vi "IRC5ControlViaOPC.vi"() -> ()   [LabVIEW 2019]
uses:
  <vilib>/OPCUA/controls/NodeId.ctl
  <vilib>/OPCUA/controls/Write Status.ctl
  <vilib>/OPCUA/controls/NodeIds.ctl
  <vilib>/OPCUA/controls/OPC UA StatusCode.ctl
  <vilib>/numeric/Random Number (Range) U64.vi
  <vilib>/numeric/sub_Random U32.vi
  <vilib>/OPCUA/client/Multiple Read Bool.vi
  <vilib>/OPCUA/client/Multiple Write Bool.vi
  <vilib>/OPCUA/NI OPC UA Client.lvlib
panel:
  in  "username/password":cluster{"username":string, "password":string}
  in  "Start":bool
  out "Color Box 45":u32(colorbox)
  out "Color Box 44":u32(colorbox)
  out "Color Box 43":u32(colorbox)
  out "Color Box 42":u32(colorbox)
  out "Color Box 41":u32(colorbox)
  out "Color Box 40":u32(colorbox)
  out "Color Box 39":u32(colorbox)
  out "Color Box 38":u32(colorbox)
  out "Color Box 37":u32(colorbox)
  out "Color Box 36":u32(colorbox)
  out "Color Box 35":u32(colorbox)
  out "Color Box 34":u32(colorbox)
  out "Color Box 33":u32(colorbox)
  out "Color Box 32":u32(colorbox)
  out "Color Box 31":u32(colorbox)
  out "Color Box 30":u32(colorbox)
  out "Color Box 29":u32(colorbox)
  out "Color Box 28":u32(colorbox)
  out "Color Box 27":u32(colorbox)
  out "Color Box 26":u32(colorbox)
  out "Color Box 25":u32(colorbox)
  out "Color Box 24":u32(colorbox)
  out "Color Box 23":u32(colorbox)
  out "Color Box 22":u32(colorbox)
  out "Color Box 21":u32(colorbox)
  out "Color Box 20":u32(colorbox)
  out "Color Box 19":u32(colorbox)
  out "Color Box 18":u32(colorbox)
  out "Color Box 12":u32(colorbox)
  out "Color Box 6":u32(colorbox)
  out "Color Box 17":u32(colorbox)
  out "Color Box 16":u32(colorbox)
  out "Color Box 15":u32(colorbox)
  out "Color Box 14":u32(colorbox)
  out "Color Box 13":u32(colorbox)
  out "Color Box 11":u32(colorbox)
  out "Color Box 10":u32(colorbox)
  out "Color Box 9":u32(colorbox)
  out "Color Box 8":u32(colorbox)
  out "Color Box 7":u32(colorbox)
  out "Color Box 5":u32(colorbox)
  out "Color Box 4":u32(colorbox)
  out "Color Box 3":u32(colorbox)
  out "Color Box 2":u32(colorbox)
  out "Color Box":u32(colorbox)
  out "Praca robota":bool
  out "element2":u32(colorbox)
  out "Układanie na palecie 3":bool
  out "Układanie na palecie 2":bool
  out "Układanie na palecie 1":bool
  out "Wrzucanie do kosza":bool
  out "Ilość elementów na palecie 1":dbl
  in  "Kolor na palecie 3":u16(ring) items=["czerwony", "zielony", "niebieski", "zółty", ""]
  in  "Kolor na palecie 2":u16(ring) items=["czerwony", "zielony", "niebieski", "zółty", ""]
  in  "Kolor na palecie 1":u16(ring) items=["czerwony", "zielony", "niebieski", "zółty", ""]
  in  "Kolor w koszu":u16(ring) items=["czerwony", "zielony", "niebieski", "zółty", ""]
  in  "milliseconds to wait 2":u32
  in  "milliseconds to wait":u32
  out "element":u32(colorbox)
  out "Ilość elementów na palecie 3":dbl
  out "Ilość elementów na palecie 2":dbl
  out "Ilość elementów w koszu":dbl
  out "Koniec przejazdu":bool
  out "Przejazd na przenośniku":bool
  out "Aktualny kolor":string
  in  "Sposób wyboru kolorów":enum32{"Losowanie", "Manualny Wybór"}(tab)
  out "Losowany kolor":string
  in  "Częstotliwość":dbl
  in  "Radio Buttons":enum32{"1", "2", "3", "4"}(radio)
  out "results":T3(array[cluster]) {"status" items=["Good"=0, "Good_SubscriptionTransferred"=2949120, "Good_CompletesAsynchronously"=3014656, "Good_Overload"=3080192, "Good_Clamped"=3145728, "Good_LocalOverride"=9830400, "Good_EntryInserted"=10616832, "Good_EntryReplaced"=10682368, "Good_NoData"=10813440, "Good_MoreData"=10878976, "Good_CommunicationEvent"=10944512, "Good_ShutdownEvent"=11010048, "Good_CallAgain"=11075584, "Good_NonCriticalTimeout"=11141120, "Good_ResultsMayBeIncomplete"=12189696, "Good_DataIgnored"=14221312, "Uncertain"=1073741824, "Uncertain_ReferenceOutOfServer"=1080819712, "Uncertain_NoCommunicationLastUsableValue"=1083113472, "Uncertain_LastUsableValue"=1083179008, "Uncertain_SubstituteValue"=1083244544, "Uncertain_InitialValue"=1083310080, "Uncertain_SensorNotAccurate"=1083375616, "Uncertain_EngineeringUnitsExceeded"=1083441152, "Uncertain_SubNormal"=1083506688, "Uncertain_DataSubNormal"=1084489728, "Uncertain_ReferenceNotDeleted"=1086062592, "Uncertain_NotAllNodesAvailable"=1086324736, "Bad"=2147483648, "Bad_UnexpectedError"=2147549184, "Bad_InternalError"=2147614720, "Bad_OutOfMemory"=2147680256, "Bad_ResourceUnavailable"=2147745792, "Bad_CommunicationError"=2147811328, "Bad_EncodingError"=2147876864, "Bad_DecodingError"=2147942400, "Bad_EncodingLimitsExceeded"=2148007936, "Bad_UnknownResponse"=2148073472, "Bad_Timeout"=2148139008, "Bad_ServiceUnsupported"=2148204544, "Bad_Shutdown"=2148270080, "Bad_ServerNotConnected"=2148335616, "Bad_ServerHalted"=2148401152, "Bad_NothingToDo"=2148466688, "Bad_TooManyOperations"=2148532224, "Bad_DataTypeIdUnknown"=2148597760, "Bad_CertificateInvalid"=2148663296, "Bad_SecurityChecksFailed"=2148728832, "Bad_CertificateTimeInvalid"=2148794368, "Bad_CertificateIssuerTimeInvalid"=2148859904, "Bad_CertificateHostNameInvalid"=2148925440, "Bad_CertificateUriInvalid"=2148990976, "Bad_CertificateUseNotAllowed"=2149056512, "Bad_CertificateIssuerUseNotAllowed"=2149122048, "Bad_CertificateUntrusted"=2149187584, "Bad_CertificateRevocationUnknown"=2149253120, "Bad_CertificateIssuerRevocationUnknown"=2149318656, "Bad_CertificateRevoked"=2149384192, "Bad_CertificateIssuerRevoked"=2149449728, "Bad_UserAccessDenied"=2149515264, "Bad_IdentityTokenInvalid"=2149580800, "Bad_IdentityTokenRejected"=2149646336, "Bad_SecureChannelIdInvalid"=2149711872, "Bad_InvalidTimestamp"=2149777408, "Bad_NonceInvalid"=2149842944, "Bad_SessionIdInvalid"=2149908480, "Bad_SessionClosed"=2149974016, "Bad_SessionNotActivated"=2150039552, "Bad_SubscriptionIdInvalid"=2150105088, "Bad_RequestHeaderInvalid"=2150236160, "Bad_TimestampsToReturnInvalid"=2150301696, "Bad_RequestCancelledByClient"=2150367232, "Bad_NoCommunication"=2150694912, "Bad_WaitingForInitialData"=2150760448, "Bad_NodeIdInvalid"=2150825984, "Bad_NodeIdUnknown"=2150891520, "Bad_AttributeIdInvalid"=2150957056, "Bad_IndexRangeInvalid"=2151022592, "Bad_IndexRangeNoData"=2151088128, "Bad_DataEncodingInvalid"=2151153664, "Bad_DataEncodingUnsupported"=2151219200, "Bad_NotReadable"=2151284736, "Bad_NotWritable"=2151350272, "Bad_OutOfRange"=2151415808, "Bad_NotSupported"=2151481344, "Bad_NotFound"=2151546880, "Bad_ObjectDeleted"=2151612416, "Bad_NotImplemented"=2151677952, "Bad_MonitoringModeInvalid"=2151743488, "Bad_MonitoredItemIdInvalid"=2151809024, "Bad_MonitoredItemFilterInvalid"=2151874560, "Bad_MonitoredItemFilterUnsupported"=2151940096, "Bad_FilterNotAllowed"=2152005632, "Bad_StructureMissing"=2152071168, "Bad_EventFilterInvalid"=2152136704, "Bad_ContentFilterInvalid"=2152202240, "Bad_FilterOperandInvalid"=2152267776, "Bad_ContinuationPointInvalid"=2152333312, "Bad_NoContinuationPoints"=2152398848, "Bad_ReferenceTypeIdInvalid"=2152464384, "Bad_BrowseDirectionInvalid"=2152529920, "Bad_NodeNotInView"=2152595456, "Bad_ServerUriInvalid"=2152660992, "Bad_ServerNameMissing"=2152726528, "Bad_DiscoveryUrlMissing"=2152792064, "Bad_SempahoreFileMissing"=2152857600, "Bad_RequestTypeInvalid"=2152923136, "Bad_SecurityModeRejected"=2152988672, "Bad_SecurityPolicyRejected"=2153054208, "Bad_TooManySessions"=2153119744, "Bad_UserSignatureInvalid"=2153185280, "Bad_ApplicationSignatureInvalid"=2153250816, "Bad_NoValidCertificates"=2153316352, "Bad_RequestCancelledByRequest"=2153381888, "Bad_ParentNodeIdInvalid"=2153447424, "Bad_ReferenceNotAllowed"=2153512960, "Bad_NodeIdRejected"=2153578496, "Bad_NodeIdExists"=2153644032, "Bad_NodeClassInvalid"=2153709568, "Bad_BrowseNameInvalid"=2153775104, "Bad_BrowseNameDuplicated"=2153840640, "Bad_NodeAttributesInvalid"=2153906176, "Bad_TypeDefinitionInvalid"=2153971712, "Bad_SourceNodeIdInvalid"=2154037248, "Bad_TargetNodeIdInvalid"=2154102784, "Bad_DuplicateReferenceNotAllowed"=2154168320, "Bad_InvalidSelfReference"=2154233856, "Bad_ReferenceLocalOnly"=2154299392, "Bad_NoDeleteRights"=2154364928, "Bad_ServerIndexInvalid"=2154430464, "Bad_ViewIdUnknown"=2154496000, "Bad_TooManyMatches"=2154627072, "Bad_QueryTooComplex"=2154692608, "Bad_NoMatch"=2154758144, "Bad_MaxAgeInvalid"=2154823680, "Bad_HistoryOperationInvalid"=2154889216, "Bad_HistoryOperationUnsupported"=2154954752, "Bad_WriteNotSupported"=2155020288, "Bad_TypeMismatch"=2155085824, "Bad_MethodInvalid"=2155151360, "Bad_ArgumentsMissing"=2155216896, "Bad_TooManySubscriptions"=2155282432, "Bad_TooManyPublishRequests"=2155347968, "Bad_NoSubscription"=2155413504, "Bad_SequenceNumberUnknown"=2155479040, "Bad_MessageNotAvailable"=2155544576, "Bad_InsufficientClientProfile"=2155610112, "Bad_TcpServerTooBusy"=2155675648, "Bad_TcpMessageTypeInvalid"=2155741184, "Bad_TcpSecureChannelUnknown"=2155806720, "Bad_TcpMessageTooLarge"=2155872256, "Bad_TcpNotEnoughResources"=2155937792, "Bad_TcpInternalError"=2156003328, "Bad_TcpEndpointUrlInvalid"=2156068864, "Bad_RequestInterrupted"=2156134400, "Bad_RequestTimeout"=2156199936, "Bad_SecureChannelClosed"=2156265472, "Bad_SecureChannelTokenUnknown"=2156331008, "Bad_SequenceNumberInvalid"=2156396544, "Bad_ConfigurationError"=2156462080, "Bad_NotConnected"=2156527616, "Bad_DeviceFailure"=2156593152, "Bad_SensorFailure"=2156658688, "Bad_OutOfService"=2156724224, "Bad_DeadbandFilterInvalid"=2156789760, "Bad_RefreshInProgress"=2157379584, "Bad_ConditionAlreadyDisabled"=2157445120, "Bad_ConditionDisabled"=2157510656, "Bad_EventIdUnknown"=2157576192, "Bad_NoData"=2157641728, "Bad_DataLost"=2157772800, "Bad_DataUnavailable"=2157838336, "Bad_EntryExists"=2157903872, "Bad_NoEntryExists"=2157969408, "Bad_TimestampNotSupported"=2158034944, "Bad_InvalidArgument"=2158690304, "Bad_ConnectionRejected"=2158755840, "Bad_Disconnect"=2158821376, "Bad_ConnectionClosed"=2158886912, "Bad_InvalidState"=2158952448, "Bad_EndOfStream"=2159017984, "Bad_NoDataAvailable"=2159083520, "Bad_WaitingForResponse"=2159149056, "Bad_OperationAbandoned"=2159214592, "Bad_ExpectedStreamToBlock"=2159280128, "Bad_WouldBlock"=2159345664, "Bad_SyntaxError"=2159411200, "Bad_MaxConnectionsReached"=2159476736, "Bad_RequestTooLarge"=2159542272, "Bad_ResponseTooLarge"=2159607808, "Bad_EventNotAcknowledgeable"=2159738880, "Bad_InvalidTimestampArgument"=2159869952, "Bad_ProtocolVersionUnsupported"=2159935488, "Bad_StateNotActive"=2160001024, "Bad_FilterOperatorInvalid"=2160132096, "Bad_FilterOperatorUnsupported"=2160197632, "Bad_FilterOperandCountMismatch"=2160263168, "Bad_FilterElementInvalid"=2160328704, "Bad_FilterLiteralInvalid"=2160394240, "Bad_IdentityChangeNotSupported"=2160459776, "Bad_NotTypeDefinition"=2160590848, "Bad_ViewTimestampInvalid"=2160656384, "Bad_ViewParameterMismatch"=2160721920, "Bad_ViewVersionInvalid"=2160787456, "Bad_ConditionAlreadyEnabled"=2160852992, "Bad_DialogNotActive"=2160918528, "Bad_DialogResponseInvalid"=2160984064, "Bad_ConditionBranchAlreadyAcked"=2161049600, "Bad_ConditionBranchAlreadyConfirmed"=2161115136, "Bad_ConditionAlreadyShelved"=2161180672, "Bad_ConditionNotShelved"=2161246208, "Bad_ShelvingTimeOutOfRange"=2161311744, "Bad_AggregateListMismatch"=2161377280, "Bad_AggregateNotSupported"=2161442816, "Bad_AggregateInvalidInputs"=2161508352, "Bad_BoundNotFound"=2161573888, "Bad_BoundNotSupported"=2161639424, "Bad_AggregateConfigurationRejected"=2161770496, "Bad_TooManyMonitoredItems"=2161836032]}
  in  "node IDs":T4
  in  "requests":T6(array[cluster]) {"node status" items=["Good"=0, "Uncertain"=1073741824, "Uncertain_InitialValue"=1083310080, "Uncertain_LastUsableValue"=1083179008, "Uncertain_SensorNotAccurate"=1083375616, "Uncertain_EngineeringUnitsExceeded"=1083441152, "Bad"=2147483648, "Bad_NoCommunication"=2150694912, "Bad_NotReadable"=2151284736, "Bad_NotWritable"=2151350272, "Bad_OutOfRange"=2151415808, "Bad_WaitingForInitialData"=2150760448]}
  in  "client certificate file":path
  in  "security policy":T7
  in  "stop":bool
  in  "trust any server (F)":bool
  in  "server endpoint URL":string
  # "Konfigutracja OPC CLIENT"
  # "Sterowanie procesem"
  # "Wizualizacja procesu"
  # "Paleta nr3"
  # "Sterowanie programem"
  # "Paleta nr1"
  # "Paleta nr2"
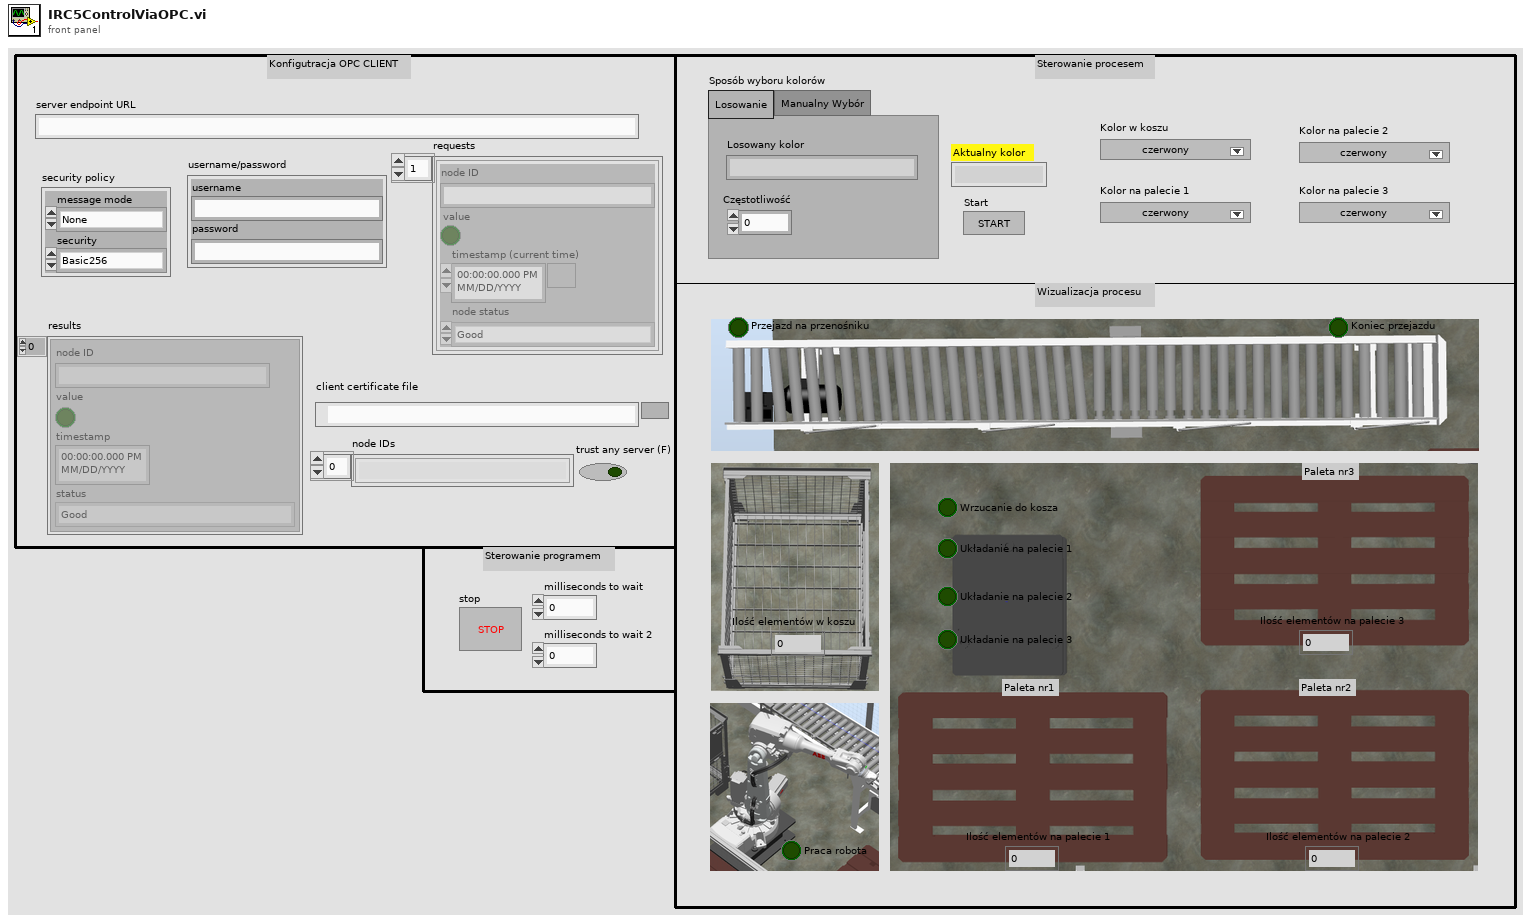
[diagram p1: front panel]
types:
  T1 = typedef "NodeId.ctl" = string
  T2 = typedef "OPC UA StatusCode.ctl" = u32
  T3 = cluster{"node ID":T1, "value ":bool, "timestamp":timestamp, "status":T2}[]
  T4 = typedef "NodeIds.ctl" = T1[]
  T5 = typedef "Write Status.ctl" = u32
  T6 = cluster{"node ID":T1, "value":bool, "timestamp (current time)":timestamp, "node status":T5}[]
  T7 = cluster{"message mode":enum16{"None", "Sign", "Sign and Encrypt"}, "security":enum16{"Basic256", "Basic128Rsa15"}}
  T8 = typedef "OPC UA Client Refnum.ctl" = refnum<k21>
  T9 = cluster{"node ID":T1, "value":bool, "timestamp (current time)":timestamp, "node status":T5}
  T10 = cluster{"node ID":T1, "Start":bool, "timestamp (current time)":timestamp, "node status":T5}
  T11 = cluster{"node ID":T1, "value ":bool, "timestamp":timestamp, "status":T2}
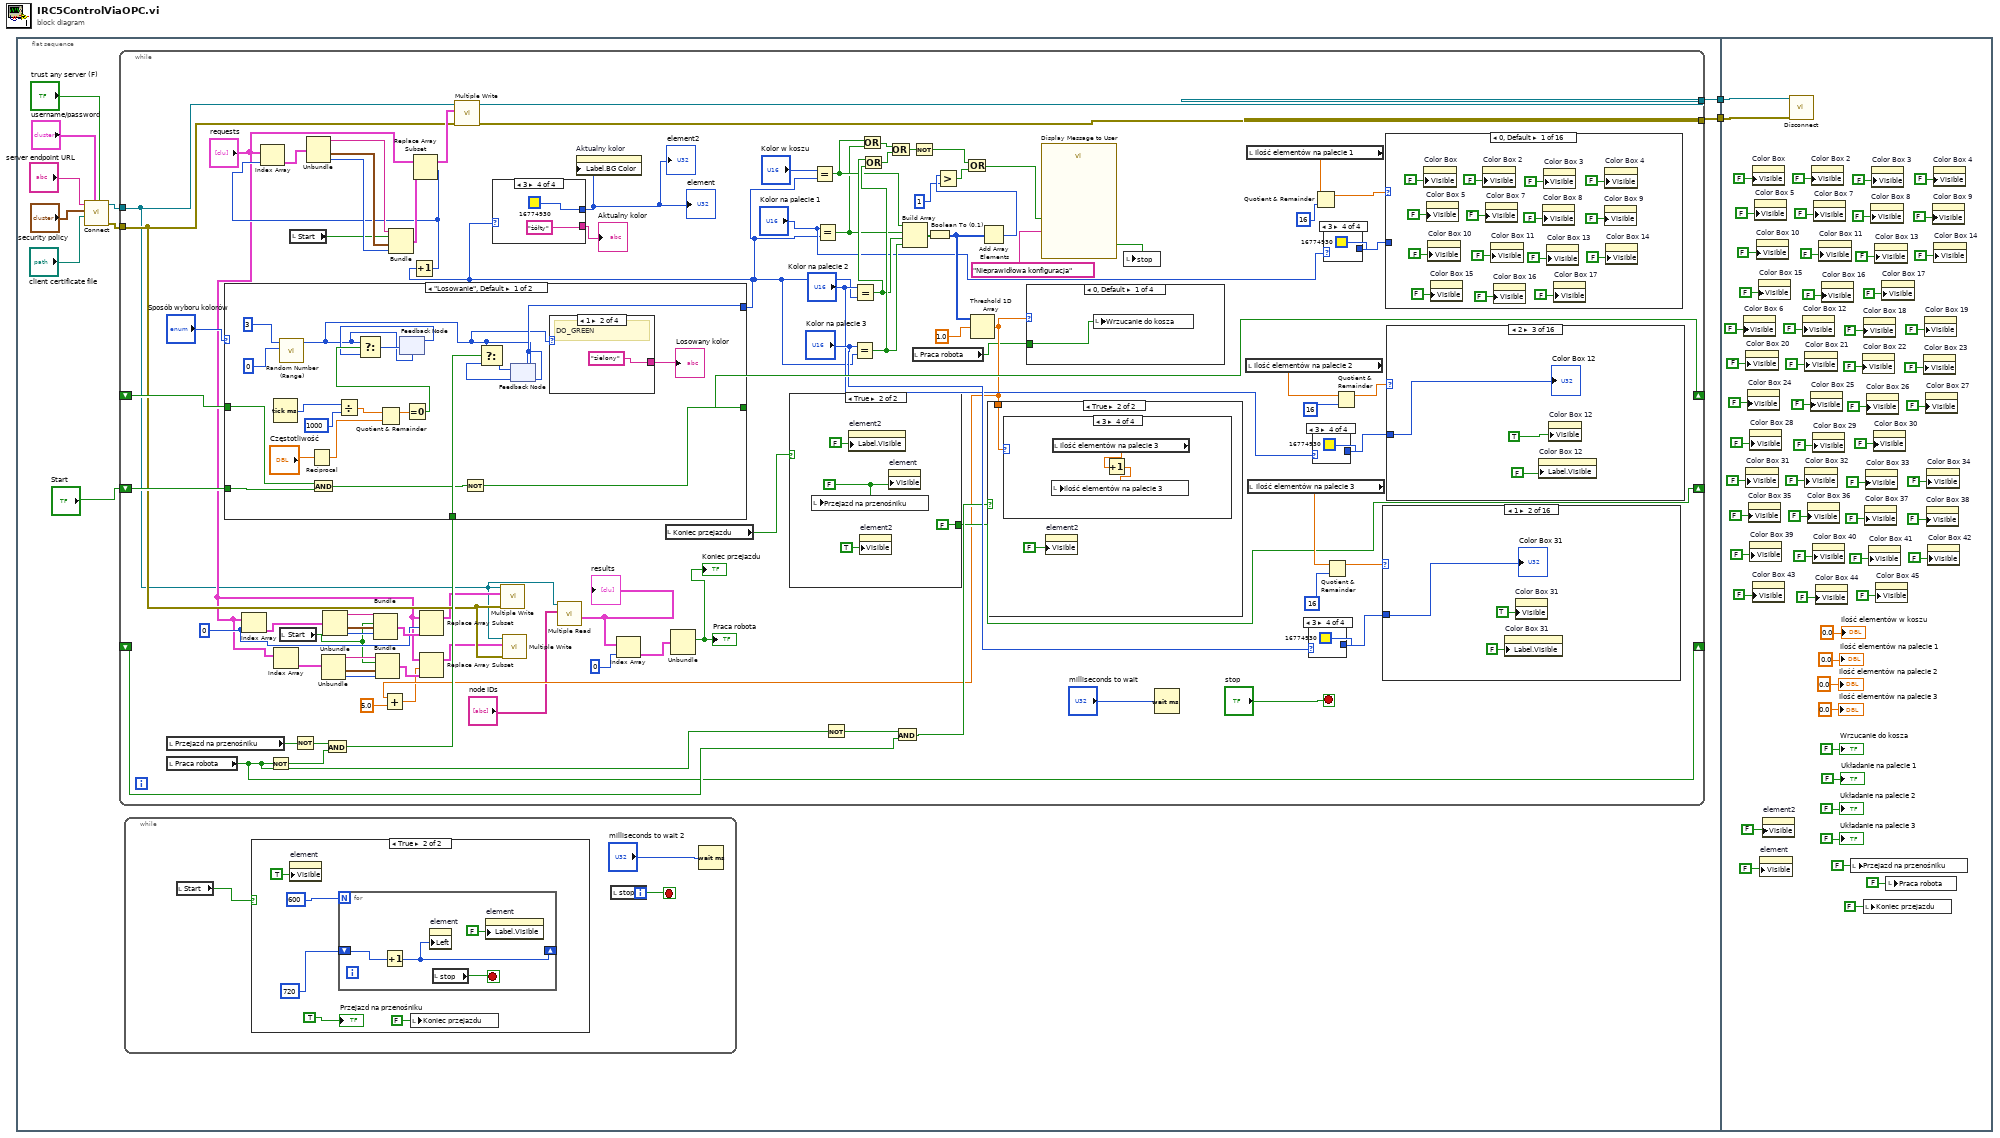
[diagram p0: block diagram]
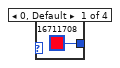
[diagram p3: hidden frame]
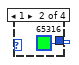
[diagram p4: hidden frame]
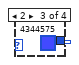
[diagram p5: hidden frame]
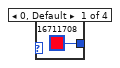
[diagram p6: hidden frame]
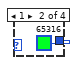
[diagram p7: hidden frame]
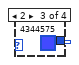
[diagram p8: hidden frame]
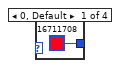
[diagram p9: hidden frame]
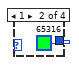
[diagram p10: hidden frame]
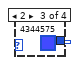
[diagram p11: hidden frame]
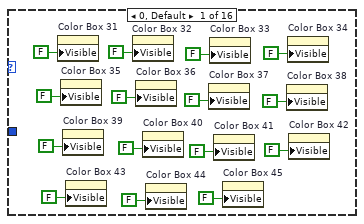
[diagram p12: hidden frame]
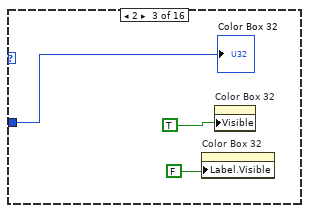
[diagram p13: hidden frame]
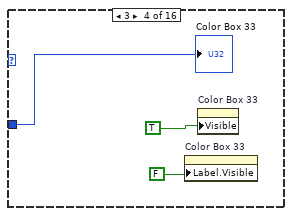
[diagram p14: hidden frame]
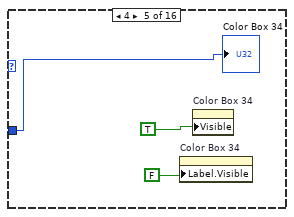
[diagram p15: hidden frame]
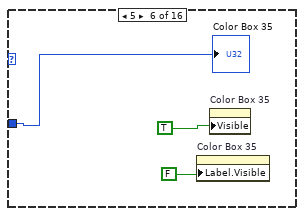
[diagram p16: hidden frame]
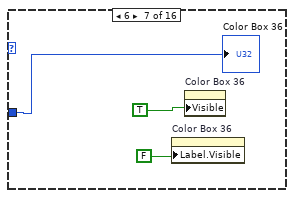
[diagram p17: hidden frame]
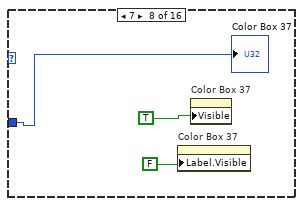
[diagram p18: hidden frame]
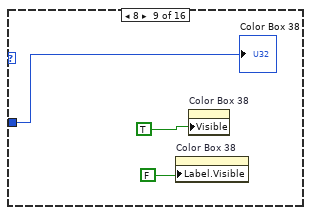
[diagram p19: hidden frame]
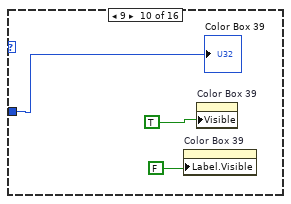
[diagram p20: hidden frame]
diagram:
  n1 = flat-sequence {
    tunnel: [w9] -> w2
    tunnel: [w8] -> w1
    tunnel: w2 -> [w363]
    tunnel: w1 -> [w364]
    frame #0 {
      n2 = call <vilib>:"Connect.vi"("trust any server (F)"="trust any server (F)", "username/password"="username/password", "client certificate file"="client certificate file", "security policy"="security policy", "server endpoint URL"="server endpoint URL") -> ("error out"=w10:errorcluster, "OPC UA client refnum out"=w11:T8)  [unwired: 4 in, 1 out]
      n3 = while {
        tunnel: w11 -> [w25]
        tunnel: w10 -> [w51]
        tunnel: [w112] -> w9
        tunnel: [w111] -> w8
        shift-right: [w75] -> _
        shift-left: _ -> [w103]
        shift-right: [w55] -> _
        shift-left: _ -> [w56]
        shift-right: [w58] -> _
        shift-left: "Start" -> [w57]
        stop <- "stop" stop-if-true
        w40 = 0 ("index")
        n4 = local read "Przejazd na przenośniku"() -> (w80:bool)
        n5 = local read "Praca robota"() -> (w55:bool)
        n6 = Index Array(array="requests", index=w40) -> (element=w50:T9)
        n7 = Not(x=w55) -> (.not. x?=w68:bool)
        n8 = Index Array(array="requests") -> (element=w48:T9)  [unwired: 1 in]
        n9 = local read "Start"() -> (w39:bool)
        n10 = local read "Start"() -> (w49:bool)
        n11 = Not(x=w80) -> (.not. x?=w79:bool)
        n12 = Unbundle(w48) -> ("node ID"=w47:T1, "timestamp (current time)"=w46:timestamp, "node status"=w45:T5)  [unwired: 1 out]
        n13 = Unbundle(w50) -> ("node ID"=w44:T1, "timestamp (current time)"=w43:timestamp, "node status"=w42:T5)  [unwired: 1 out]
        n14 = And(x=w79, y=w68) -> (x .and. y?=w59:bool)
        n15 = case shown="\"Losowanie\", Default" "Sposób wyboru kolorów" {
          tunnel: [w347 w358] -> w53
          tunnel: [w345 w361] -> w75
          tunnel: w103 -> [w346 w362]
          tunnel: w57 -> [w336 w356]
          tunnel: w59 -> [w335 _]
          frame "Losowanie", Default {
            n16 = Tick Count (ms)() -> (millisecond timer value=w343:u32)
            n17 = call-poly <vilib>:"Random Number (Range).vi"("lower bound (0)"=u64 0, "upper bound (100)"=u64 3) -> ("number"=w332:u64)  [unwired: 9 in]
            n18 = Reciprocal(x="Częstotliwość") -> (1/x=w341:dbl)
            n19 = And(x=w346, y=w336) -> (x .and. y?=w334:bool)
            n20 = Divide(x=w343, y=1000) -> (x/y=w344:dbl)
            n21 = Quotient & Remainder(x=w344, y=w341) -> (x-y*floor(x/y)=w339:dbl)  [unwired: 1 out]
            n22 = feedback #1(w332) -> (w333:u64)
            n23 = Equal To 0?(x=w339) -> (x = 0?=w338:bool)
            n24 = Select(t=w332, s=w338, f=w333) -> (s? t:f=w337:u64)
            n25 = feedback-in #1(w337) -> ()
            n26 = Not(x=w334) -> (.not. x?=w345:bool)
            n27 = feedback #2(w332) -> (w347:u64)
            n28 = Select(t=w332, s=w335, f=w347) -> (s? t:f=w349:u64)
            n29 = feedback-in #2(w349) -> ()
            n30 = case shown="1" w332 {
              tunnel: ["czerwony" "zielony" "niebieski" "żółty"] -> w348
              frame 0, Default {
                # "DO_RED"
              }
              frame 1 {
                # "DO_GREEN"
              }
              frame 2 {
                # "DO_BLUE"
              }
              frame 3 {
                # "DO_YELLOW"
              }
            }
            "Losowany kolor" <- w348
          }
          frame "Manualny Wybór" {
            n31 = And(x=w362, y=w356) -> (x .and. y?=w360:bool)
            n32 = feedback #3("Radio Buttons") -> (w359:enum32{"1", "2", "3", "4"})
            n33 = Select(t="Radio Buttons", s=w360, f=w359) -> (s? t:f=w358:enum32{"1", "2", "3", "4"})
            n34 = feedback-in #3(w358) -> ()
            n35 = Not(x=w356) -> (.not. x?=w361:bool)
          }
        }
        n36 = Bundle("node ID"=w44, "Start"=w39, "timestamp (current time)"=w43, "node status"=w42) -> (w41:T10)  [unwired: 1 in]
        n37 = Bundle("node ID"=w47, "Start"=w39, "timestamp (current time)"=w46, "node status"=w45) -> (w38:T10)  [unwired: 1 in]
        n38 = Increment(x=w53) -> (x+1=w52:u64)
        n39 = Index Array(array="requests", index=w52) -> (element=w110:T9)
        n40 = Unbundle(w110) -> ("node ID"=w107:T1, "timestamp (current time)"=w109:timestamp, "node status"=w108:T5)  [unwired: 1 out]
        n41 = Bundle("node ID"=w107, "Start"=w49, "timestamp (current time)"=w109, "node status"=w108) -> (w106:T10)  [unwired: 1 in]
        n42 = Replace Array Subset(array="requests", new element=w106, index=w52) -> (w105:T6)
        n43 = Replace Array Subset(array="requests", new element=w41, index=w40) -> (w32:T6)
        n44 = call-poly <vilib>:"Multiple Write.vi"("error in (no error)"=w51, "requests"=w105, "OPC UA client refnum in"=w25) -> ("error out"=w111:errorcluster, "OPC UA client refnum out"=w112:T8)  [unwired: 5 in, 2 out]
        n45 = case shown="3" w53 {
          tunnel: [u32 16711708 ("Caption.Colors:FG Color") u32 65316 ("Caption.Colors:FG Color") u32 4344575 ("Caption.Colors:FG Color") u32 16774930 ("Caption.Colors:FG Color")] -> w67
          tunnel: ["czerwony" "zielony" "niebieski" "żółty"] -> w102
          frame 0, Default {
          }
          frame 1 {
          }
          frame 2 {
          }
          frame 3 {
          }
        }
        "Aktualny kolor" <- w102
        "element" <- w67
        "element2" <- w67
        n46 = call-poly <vilib>:"Multiple Write.vi"("error in (no error)"=w51, "requests"=w32, "OPC UA client refnum in"=w25) -> ()  [unwired: 5 in, 4 out]
        n47 = call-poly <vilib>:"Multiple Read.vi"("node IDs"="node IDs", "OPC UA client refnum in"=w25) -> ("results"=w29:T3)  [unwired: 6 in, 3 out]
        "results" <- w29
        n48 = property on="Aktualny kolor" class="Str"("Label.BG Color"=w67) -> ()  [unwired: 2 in, 2 out]
        n49 = Index Array(array=w29, index=0) -> (element=w28:T11)
        n50 = local read "Koniec przejazdu"() -> (w81:bool)
        n51 = Unbundle(w28) -> ("value"=→"Koniec przejazdu" →"Praca robota":bool)  [unwired: 3 out]
        n52 = case shown="True" w81 {
          tunnel: [TRUE FALSE] -> w58
          frame False {
          }
          frame True {
            w318 = FALSE ("Visible")
            n53 = local write "Przejazd na przenośniku"(w318) -> ()
            n54 = property on="element2" class="ColBox"("Label.Visible"=FALSE ("Visible")) -> ()  [unwired: 2 in, 2 out]
            n55 = property on="element2" class="ColBox"("Visible"=TRUE) -> ()  [unwired: 2 in, 2 out]
            n56 = property on="element" class="ColBox"("Visible"=w318) -> ()  [unwired: 2 in, 2 out]
          }
        }
        n57 = Equal?(x="Kolor w koszu", y=w53) -> (x = y?=w85:bool)
        n58 = Equal?(x="Kolor na palecie 1", y=w53) -> (x = y?=w84:bool)
        n59 = Not(x=w55) -> (.not. x?=w54:bool)
        n60 = Equal?(x="Kolor na palecie 3", y=w53) -> (x = y?=w96:bool)
        n61 = Equal?(x="Kolor na palecie 2", y=w53) -> (x = y?=w95:bool)
        n62 = Or(x=w85, y=w84) -> (x .or. y?=w98:bool)
        n63 = Or(x=w95, y=w96) -> (x .or. y?=w97:bool)
        n64 = Or(x=w98, y=w97) -> (x .or. y?=w94:bool)
        n65 = And(x=w54, y=w56) -> (x .and. y?=w60:bool)
        n66 = Build Array(w85, w84, w95, w96) -> (w93:bool[])
        n67 = Not(x=w94) -> (.not. x?=w92:bool)
        n68 = local read "Praca robota"() -> (w26:bool)
        n69 = Boolean To (0,1)(Boolean=w93) -> (0, 1=w83:i16[])
        n70 = Threshold 1D Array(2:1.0 ("threshold y"), 3:w83) -> (0:w37:dbl)  [unwired: 1 in]
        n71 = Add(x=w37, y=5.0) -> (x+y=w34:dbl)
        n72 = Replace Array Subset(array="requests", new element=w38, index=w34) -> (w33:T6)
        n73 = call-poly <vilib>:"Multiple Write.vi"("error in (no error)"=w51, "requests"=w33, "OPC UA client refnum in"=w25) -> ()  [unwired: 5 in, 4 out]
        n74 = Add Array Elements(numeric array=w83) -> (sum=w90:i16)
        n75 = Greater?(x=w90, y=1) -> (0:w91:bool)
        n76 = Or(x=w92, y=w91) -> (x .or. y?=w88:bool)
        n77 = case shown="True" w60 {
          tunnel: w37 -> [_ w306]
          frame False {
          }
          frame True {
            n78 = case shown="3" w306 {
              frame 0, Default {
                n79 = local read "Ilość elementów w koszu"() -> (w308:dbl)
                n80 = Increment(x=w308) -> (x+1=w307:dbl)
                n81 = local write "Ilość elementów w koszu"(w307) -> ()
              }
              frame 1 {
                n82 = local read "Ilość elementów na palecie 1"() -> (w310:dbl)
                n83 = Increment(x=w310) -> (x+1=w309:dbl)
                n84 = local write "Ilość elementów na palecie 1"(w309) -> ()
              }
              frame 2 {
                n85 = local read "Ilość elementów na palecie 2"() -> (w312:dbl)
                n86 = Increment(x=w312) -> (x+1=w311:dbl)
                n87 = local write "Ilość elementów na palecie 2"(w311) -> ()
              }
              frame 3 {
                n88 = local read "Ilość elementów na palecie 3"() -> (w314:dbl)
                n89 = Increment(x=w314) -> (x+1=w313:dbl)
                n90 = local write "Ilość elementów na palecie 3"(w313) -> ()
              }
            }
            n91 = property on="element2" class="ColBox"("Visible"=FALSE) -> ()  [unwired: 2 in, 2 out]
          }
        }
        n92 = case shown="0, Default" w37 {
          tunnel: w26 -> [w320 w321 w322 w323]
          frame 0, Default {
            n93 = local write "Wrzucanie do kosza"(w320) -> ()
          }
          frame 1 {
            n94 = local write "Układanie na palecie 1"(w321) -> ()
          }
          frame 2 {
            n95 = local write "Układanie na palecie 2"(w322) -> ()
          }
          frame 3 {
            n96 = local write "Układanie na palecie 3"(w323) -> ()
          }
        }
        n97 = call "Display Message to User"("Enable"=w88, "Message"="Nieprawidłowa konfiguracja") -> ("OK"=w86:bool)  [unwired: 8 in, 1 out]
        n98 = local write "stop"(w86) -> ()
        n99 = Wait (ms)(milliseconds to wait="milliseconds to wait") -> ()  [unwired: 1 out]
        n100 = local read "Ilość elementów na palecie 2"() -> (w72:dbl)
        n101 = local read "Ilość elementów na palecie 1"() -> (w76:dbl)
        n102 = local read "Ilość elementów na palecie 3"() -> (w71:dbl)
        n103 = case shown="3" "Kolor na palecie 3" {
          tunnel: [u32 16711708 ("Caption.Colors:FG Color") u32 65316 ("Caption.Colors:FG Color") u32 4344575 ("Caption.Colors:FG Color") u32 16774930 ("Caption.Colors:FG Color")] -> w65
          frame 0, Default {
          }
          frame 1 {
          }
          frame 2 {
          }
          frame 3 {
          }
        }
        n104 = case shown="3" "Kolor na palecie 2" {
          tunnel: [u32 16711708 ("Caption.Colors:FG Color") u32 65316 ("Caption.Colors:FG Color") u32 4344575 ("Caption.Colors:FG Color") u32 16774930 ("Caption.Colors:FG Color")] -> w61
          frame 0, Default {
          }
          frame 1 {
          }
          frame 2 {
          }
          frame 3 {
          }
        }
        n105 = Quotient & Remainder(x=w76, y=16) -> (x-y*floor(x/y)=w77:dbl)  [unwired: 1 out]
        n106 = case shown="3" "Kolor na palecie 1" {
          tunnel: [u32 16711708 ("Caption.Colors:FG Color") u32 65316 ("Caption.Colors:FG Color") u32 4344575 ("Caption.Colors:FG Color") u32 16774930 ("Caption.Colors:FG Color")] -> w64
          frame 0, Default {
          }
          frame 1 {
          }
          frame 2 {
          }
          frame 3 {
          }
        }
        n107 = Quotient & Remainder(x=w71, y=16) -> (x-y*floor(x/y)=w69:dbl)  [unwired: 1 out]
        n108 = Quotient & Remainder(x=w72, y=16) -> (x-y*floor(x/y)=w70:dbl)  [unwired: 1 out]
        n109 = case shown="1" w69 {
          tunnel: w65 -> [_ w142 w145 w148 w151 w154 w157 w160 w163 w166 w169 w172 w175 w178 w181 w184]
          frame 0, Default {
            n110 = property on="Color Box 31" class="ColBox"("Visible"=FALSE) -> ()  [unwired: 2 in, 2 out]
            n111 = property on="Color Box 35" class="ColBox"("Visible"=FALSE) -> ()  [unwired: 2 in, 2 out]
            n112 = property on="Color Box 39" class="ColBox"("Visible"=FALSE) -> ()  [unwired: 2 in, 2 out]
            n113 = property on="Color Box 43" class="ColBox"("Visible"=FALSE) -> ()  [unwired: 2 in, 2 out]
            n114 = property on="Color Box 32" class="ColBox"("Visible"=FALSE) -> ()  [unwired: 2 in, 2 out]
            n115 = property on="Color Box 36" class="ColBox"("Visible"=FALSE) -> ()  [unwired: 2 in, 2 out]
            n116 = property on="Color Box 40" class="ColBox"("Visible"=FALSE) -> ()  [unwired: 2 in, 2 out]
            n117 = property on="Color Box 44" class="ColBox"("Visible"=FALSE) -> ()  [unwired: 2 in, 2 out]
            n118 = property on="Color Box 37" class="ColBox"("Visible"=FALSE) -> ()  [unwired: 2 in, 2 out]
            n119 = property on="Color Box 33" class="ColBox"("Visible"=FALSE) -> ()  [unwired: 2 in, 2 out]
            n120 = property on="Color Box 41" class="ColBox"("Visible"=FALSE) -> ()  [unwired: 2 in, 2 out]
            n121 = property on="Color Box 45" class="ColBox"("Visible"=FALSE) -> ()  [unwired: 2 in, 2 out]
            n122 = property on="Color Box 38" class="ColBox"("Visible"=FALSE) -> ()  [unwired: 2 in, 2 out]
            n123 = property on="Color Box 34" class="ColBox"("Visible"=FALSE) -> ()  [unwired: 2 in, 2 out]
            n124 = property on="Color Box 42" class="ColBox"("Visible"=FALSE) -> ()  [unwired: 2 in, 2 out]
          }
          frame 1 {
            n125 = property on="Color Box 31" class="ColBox"("Label.Visible"=FALSE) -> ()  [unwired: 2 in, 2 out]
            n126 = property on="Color Box 31" class="ColBox"("Visible"=TRUE) -> ()  [unwired: 2 in, 2 out]
            "Color Box 31" <- w142
          }
          frame 2 {
            n127 = property on="Color Box 32" class="ColBox"("Label.Visible"=FALSE) -> ()  [unwired: 2 in, 2 out]
            n128 = property on="Color Box 32" class="ColBox"("Visible"=TRUE) -> ()  [unwired: 2 in, 2 out]
            "Color Box 32" <- w145
          }
          frame 3 {
            n129 = property on="Color Box 33" class="ColBox"("Label.Visible"=FALSE) -> ()  [unwired: 2 in, 2 out]
            n130 = property on="Color Box 33" class="ColBox"("Visible"=TRUE) -> ()  [unwired: 2 in, 2 out]
            "Color Box 33" <- w148
          }
          frame 4 {
            n131 = property on="Color Box 34" class="ColBox"("Label.Visible"=FALSE) -> ()  [unwired: 2 in, 2 out]
            n132 = property on="Color Box 34" class="ColBox"("Visible"=TRUE) -> ()  [unwired: 2 in, 2 out]
            "Color Box 34" <- w151
          }
          frame 5 {
            n133 = property on="Color Box 35" class="ColBox"("Label.Visible"=FALSE) -> ()  [unwired: 2 in, 2 out]
            n134 = property on="Color Box 35" class="ColBox"("Visible"=TRUE) -> ()  [unwired: 2 in, 2 out]
            "Color Box 35" <- w154
          }
          frame 6 {
            n135 = property on="Color Box 36" class="ColBox"("Label.Visible"=FALSE) -> ()  [unwired: 2 in, 2 out]
            n136 = property on="Color Box 36" class="ColBox"("Visible"=TRUE) -> ()  [unwired: 2 in, 2 out]
            "Color Box 36" <- w157
          }
          frame 7 {
            n137 = property on="Color Box 37" class="ColBox"("Label.Visible"=FALSE) -> ()  [unwired: 2 in, 2 out]
            n138 = property on="Color Box 37" class="ColBox"("Visible"=TRUE) -> ()  [unwired: 2 in, 2 out]
            "Color Box 37" <- w160
          }
          frame 8 {
            n139 = property on="Color Box 38" class="ColBox"("Label.Visible"=FALSE) -> ()  [unwired: 2 in, 2 out]
            n140 = property on="Color Box 38" class="ColBox"("Visible"=TRUE) -> ()  [unwired: 2 in, 2 out]
            "Color Box 38" <- w163
          }
          frame 9 {
            n141 = property on="Color Box 39" class="ColBox"("Label.Visible"=FALSE) -> ()  [unwired: 2 in, 2 out]
            n142 = property on="Color Box 39" class="ColBox"("Visible"=TRUE) -> ()  [unwired: 2 in, 2 out]
            "Color Box 39" <- w166
          }
          frame 10 {
            n143 = property on="Color Box 40" class="ColBox"("Label.Visible"=FALSE) -> ()  [unwired: 2 in, 2 out]
            n144 = property on="Color Box 40" class="ColBox"("Visible"=TRUE) -> ()  [unwired: 2 in, 2 out]
            "Color Box 40" <- w169
          }
          frame 11 {
            n145 = property on="Color Box 41" class="ColBox"("Label.Visible"=FALSE) -> ()  [unwired: 2 in, 2 out]
            n146 = property on="Color Box 41" class="ColBox"("Visible"=TRUE) -> ()  [unwired: 2 in, 2 out]
            "Color Box 41" <- w172
          }
          frame 12 {
            n147 = property on="Color Box 42" class="ColBox"("Label.Visible"=FALSE) -> ()  [unwired: 2 in, 2 out]
            n148 = property on="Color Box 42" class="ColBox"("Visible"=TRUE) -> ()  [unwired: 2 in, 2 out]
            "Color Box 42" <- w175
          }
          frame 13 {
            n149 = property on="Color Box 43" class="ColBox"("Label.Visible"=FALSE) -> ()  [unwired: 2 in, 2 out]
            n150 = property on="Color Box 43" class="ColBox"("Visible"=TRUE) -> ()  [unwired: 2 in, 2 out]
            "Color Box 43" <- w178
          }
          frame 14 {
            n151 = property on="Color Box 44" class="ColBox"("Label.Visible"=FALSE) -> ()  [unwired: 2 in, 2 out]
            n152 = property on="Color Box 44" class="ColBox"("Visible"=TRUE) -> ()  [unwired: 2 in, 2 out]
            "Color Box 44" <- w181
          }
          frame 15 {
            n153 = property on="Color Box 45" class="ColBox"("Label.Visible"=FALSE) -> ()  [unwired: 2 in, 2 out]
            n154 = property on="Color Box 45" class="ColBox"("Visible"=TRUE) -> ()  [unwired: 2 in, 2 out]
            "Color Box 45" <- w184
          }
        }
        n155 = case shown="0, Default" w77 {
          tunnel: w64 -> [_ w262 w265 w268 w271 w274 w277 w280 w283 w286 w289 w292 w295 w298 w301 w304]
          frame 0, Default {
            n156 = property on="Color Box" class="ColBox"("Visible"=FALSE) -> ()  [unwired: 2 in, 2 out]
            n157 = property on="Color Box 5" class="ColBox"("Visible"=FALSE) -> ()  [unwired: 2 in, 2 out]
            n158 = property on="Color Box 10" class="ColBox"("Visible"=FALSE) -> ()  [unwired: 2 in, 2 out]
            n159 = property on="Color Box 15" class="ColBox"("Visible"=FALSE) -> ()  [unwired: 2 in, 2 out]
            n160 = property on="Color Box 2" class="ColBox"("Visible"=FALSE) -> ()  [unwired: 2 in, 2 out]
            n161 = property on="Color Box 7" class="ColBox"("Visible"=FALSE) -> ()  [unwired: 2 in, 2 out]
            n162 = property on="Color Box 11" class="ColBox"("Visible"=FALSE) -> ()  [unwired: 2 in, 2 out]
            n163 = property on="Color Box 16" class="ColBox"("Visible"=FALSE) -> ()  [unwired: 2 in, 2 out]
            n164 = property on="Color Box 8" class="ColBox"("Visible"=FALSE) -> ()  [unwired: 2 in, 2 out]
            n165 = property on="Color Box 3" class="ColBox"("Visible"=FALSE) -> ()  [unwired: 2 in, 2 out]
            n166 = property on="Color Box 13" class="ColBox"("Visible"=FALSE) -> ()  [unwired: 2 in, 2 out]
            n167 = property on="Color Box 17" class="ColBox"("Visible"=FALSE) -> ()  [unwired: 2 in, 2 out]
            n168 = property on="Color Box 9" class="ColBox"("Visible"=FALSE) -> ()  [unwired: 2 in, 2 out]
            n169 = property on="Color Box 4" class="ColBox"("Visible"=FALSE) -> ()  [unwired: 2 in, 2 out]
            n170 = property on="Color Box 14" class="ColBox"("Visible"=FALSE) -> ()  [unwired: 2 in, 2 out]
          }
          frame 1 {
            n171 = property on="Color Box" class="ColBox"("Label.Visible"=FALSE) -> ()  [unwired: 2 in, 2 out]
            n172 = property on="Color Box" class="ColBox"("Visible"=TRUE) -> ()  [unwired: 2 in, 2 out]
            "Color Box" <- w262
          }
          frame 2 {
            n173 = property on="Color Box 2" class="ColBox"("Label.Visible"=FALSE) -> ()  [unwired: 2 in, 2 out]
            n174 = property on="Color Box 2" class="ColBox"("Visible"=TRUE) -> ()  [unwired: 2 in, 2 out]
            "Color Box 2" <- w265
          }
          frame 3 {
            n175 = property on="Color Box 3" class="ColBox"("Label.Visible"=FALSE) -> ()  [unwired: 2 in, 2 out]
            n176 = property on="Color Box 3" class="ColBox"("Visible"=TRUE) -> ()  [unwired: 2 in, 2 out]
            "Color Box 3" <- w268
          }
          frame 4 {
            n177 = property on="Color Box 4" class="ColBox"("Label.Visible"=FALSE) -> ()  [unwired: 2 in, 2 out]
            n178 = property on="Color Box 4" class="ColBox"("Visible"=TRUE) -> ()  [unwired: 2 in, 2 out]
            "Color Box 4" <- w271
          }
          frame 5 {
            n179 = property on="Color Box 5" class="ColBox"("Label.Visible"=FALSE) -> ()  [unwired: 2 in, 2 out]
            n180 = property on="Color Box 5" class="ColBox"("Visible"=TRUE) -> ()  [unwired: 2 in, 2 out]
            "Color Box 5" <- w274
          }
          frame 6 {
            n181 = property on="Color Box 7" class="ColBox"("Label.Visible"=FALSE) -> ()  [unwired: 2 in, 2 out]
            n182 = property on="Color Box 7" class="ColBox"("Visible"=TRUE) -> ()  [unwired: 2 in, 2 out]
            "Color Box 7" <- w277
          }
          frame 7 {
            n183 = property on="Color Box 8" class="ColBox"("Label.Visible"=FALSE) -> ()  [unwired: 2 in, 2 out]
            n184 = property on="Color Box 8" class="ColBox"("Visible"=TRUE) -> ()  [unwired: 2 in, 2 out]
            "Color Box 8" <- w280
          }
          frame 8 {
            n185 = property on="Color Box 9" class="ColBox"("Label.Visible"=FALSE) -> ()  [unwired: 2 in, 2 out]
            n186 = property on="Color Box 9" class="ColBox"("Visible"=TRUE) -> ()  [unwired: 2 in, 2 out]
            "Color Box 9" <- w283
          }
          frame 9 {
            n187 = property on="Color Box 10" class="ColBox"("Label.Visible"=FALSE) -> ()  [unwired: 2 in, 2 out]
            n188 = property on="Color Box 10" class="ColBox"("Visible"=TRUE) -> ()  [unwired: 2 in, 2 out]
            "Color Box 10" <- w286
          }
          frame 10 {
            n189 = property on="Color Box 11" class="ColBox"("Label.Visible"=FALSE) -> ()  [unwired: 2 in, 2 out]
            n190 = property on="Color Box 11" class="ColBox"("Visible"=TRUE) -> ()  [unwired: 2 in, 2 out]
            "Color Box 11" <- w289
          }
          frame 11 {
            n191 = property on="Color Box 13" class="ColBox"("Label.Visible"=FALSE) -> ()  [unwired: 2 in, 2 out]
            n192 = property on="Color Box 13" class="ColBox"("Visible"=TRUE) -> ()  [unwired: 2 in, 2 out]
            "Color Box 13" <- w292
          }
          frame 12 {
            n193 = property on="Color Box 14" class="ColBox"("Label.Visible"=FALSE) -> ()  [unwired: 2 in, 2 out]
            n194 = property on="Color Box 14" class="ColBox"("Visible"=TRUE) -> ()  [unwired: 2 in, 2 out]
            "Color Box 14" <- w295
          }
          frame 13 {
            n195 = property on="Color Box 15" class="ColBox"("Label.Visible"=FALSE) -> ()  [unwired: 2 in, 2 out]
            n196 = property on="Color Box 15" class="ColBox"("Visible"=TRUE) -> ()  [unwired: 2 in, 2 out]
            "Color Box 15" <- w298
          }
          frame 14 {
            n197 = property on="Color Box 16" class="ColBox"("Label.Visible"=FALSE) -> ()  [unwired: 2 in, 2 out]
            n198 = property on="Color Box 16" class="ColBox"("Visible"=TRUE) -> ()  [unwired: 2 in, 2 out]
            "Color Box 16" <- w301
          }
          frame 15 {
            n199 = property on="Color Box 17" class="ColBox"("Label.Visible"=FALSE) -> ()  [unwired: 2 in, 2 out]
            n200 = property on="Color Box 17" class="ColBox"("Visible"=TRUE) -> ()  [unwired: 2 in, 2 out]
            "Color Box 17" <- w304
          }
        }
        n201 = case shown="2" w70 {
          tunnel: w61 -> [_ w202 w205 w208 w211 w214 w217 w220 w223 w226 w229 w232 w235 w238 w241 w244]
          frame 0, Default {
            n202 = property on="Color Box 6" class="ColBox"("Visible"=FALSE) -> ()  [unwired: 2 in, 2 out]
            n203 = property on="Color Box 20" class="ColBox"("Visible"=FALSE) -> ()  [unwired: 2 in, 2 out]
            n204 = property on="Color Box 24" class="ColBox"("Visible"=FALSE) -> ()  [unwired: 2 in, 2 out]
            n205 = property on="Color Box 28" class="ColBox"("Visible"=FALSE) -> ()  [unwired: 2 in, 2 out]
            n206 = property on="Color Box 12" class="ColBox"("Visible"=FALSE) -> ()  [unwired: 2 in, 2 out]
            n207 = property on="Color Box 21" class="ColBox"("Visible"=FALSE) -> ()  [unwired: 2 in, 2 out]
            n208 = property on="Color Box 25" class="ColBox"("Visible"=FALSE) -> ()  [unwired: 2 in, 2 out]
            n209 = property on="Color Box 29" class="ColBox"("Visible"=FALSE) -> ()  [unwired: 2 in, 2 out]
            n210 = property on="Color Box 22" class="ColBox"("Visible"=FALSE) -> ()  [unwired: 2 in, 2 out]
            n211 = property on="Color Box 18" class="ColBox"("Visible"=FALSE) -> ()  [unwired: 2 in, 2 out]
            n212 = property on="Color Box 26" class="ColBox"("Visible"=FALSE) -> ()  [unwired: 2 in, 2 out]
            n213 = property on="Color Box 30" class="ColBox"("Visible"=FALSE) -> ()  [unwired: 2 in, 2 out]
            n214 = property on="Color Box 23" class="ColBox"("Visible"=FALSE) -> ()  [unwired: 2 in, 2 out]
            n215 = property on="Color Box 19" class="ColBox"("Visible"=FALSE) -> ()  [unwired: 2 in, 2 out]
            n216 = property on="Color Box 27" class="ColBox"("Visible"=FALSE) -> ()  [unwired: 2 in, 2 out]
          }
          frame 1 {
            n217 = property on="Color Box 6" class="ColBox"("Label.Visible"=FALSE) -> ()  [unwired: 2 in, 2 out]
            n218 = property on="Color Box 6" class="ColBox"("Visible"=TRUE) -> ()  [unwired: 2 in, 2 out]
            "Color Box 6" <- w202
          }
          frame 2 {
            n219 = property on="Color Box 12" class="ColBox"("Label.Visible"=FALSE) -> ()  [unwired: 2 in, 2 out]
            n220 = property on="Color Box 12" class="ColBox"("Visible"=TRUE) -> ()  [unwired: 2 in, 2 out]
            "Color Box 12" <- w205
          }
          frame 3 {
            n221 = property on="Color Box 18" class="ColBox"("Label.Visible"=FALSE) -> ()  [unwired: 2 in, 2 out]
            n222 = property on="Color Box 18" class="ColBox"("Visible"=TRUE) -> ()  [unwired: 2 in, 2 out]
            "Color Box 18" <- w208
          }
          frame 4 {
            n223 = property on="Color Box 19" class="ColBox"("Label.Visible"=FALSE) -> ()  [unwired: 2 in, 2 out]
            n224 = property on="Color Box 19" class="ColBox"("Visible"=TRUE) -> ()  [unwired: 2 in, 2 out]
            "Color Box 19" <- w211
          }
          frame 5 {
            n225 = property on="Color Box 20" class="ColBox"("Label.Visible"=FALSE) -> ()  [unwired: 2 in, 2 out]
            n226 = property on="Color Box 20" class="ColBox"("Visible"=TRUE) -> ()  [unwired: 2 in, 2 out]
            "Color Box 20" <- w214
          }
          frame 6 {
            n227 = property on="Color Box 21" class="ColBox"("Label.Visible"=FALSE) -> ()  [unwired: 2 in, 2 out]
            n228 = property on="Color Box 21" class="ColBox"("Visible"=TRUE) -> ()  [unwired: 2 in, 2 out]
            "Color Box 21" <- w217
          }
          frame 7 {
            n229 = property on="Color Box 22" class="ColBox"("Label.Visible"=FALSE) -> ()  [unwired: 2 in, 2 out]
            n230 = property on="Color Box 22" class="ColBox"("Visible"=TRUE) -> ()  [unwired: 2 in, 2 out]
            "Color Box 22" <- w220
          }
          frame 8 {
            n231 = property on="Color Box 23" class="ColBox"("Label.Visible"=FALSE) -> ()  [unwired: 2 in, 2 out]
            n232 = property on="Color Box 23" class="ColBox"("Visible"=TRUE) -> ()  [unwired: 2 in, 2 out]
            "Color Box 23" <- w223
          }
          frame 9 {
            n233 = property on="Color Box 24" class="ColBox"("Label.Visible"=FALSE) -> ()  [unwired: 2 in, 2 out]
            n234 = property on="Color Box 24" class="ColBox"("Visible"=TRUE) -> ()  [unwired: 2 in, 2 out]
            "Color Box 24" <- w226
          }
          frame 10 {
            n235 = property on="Color Box 25" class="ColBox"("Label.Visible"=FALSE) -> ()  [unwired: 2 in, 2 out]
            n236 = property on="Color Box 25" class="ColBox"("Visible"=TRUE) -> ()  [unwired: 2 in, 2 out]
            "Color Box 25" <- w229
          }
          frame 11 {
            n237 = property on="Color Box 26" class="ColBox"("Label.Visible"=FALSE) -> ()  [unwired: 2 in, 2 out]
            n238 = property on="Color Box 26" class="ColBox"("Visible"=TRUE) -> ()  [unwired: 2 in, 2 out]
            "Color Box 26" <- w232
          }
          frame 12 {
            n239 = property on="Color Box 27" class="ColBox"("Label.Visible"=FALSE) -> ()  [unwired: 2 in, 2 out]
            n240 = property on="Color Box 27" class="ColBox"("Visible"=TRUE) -> ()  [unwired: 2 in, 2 out]
            "Color Box 27" <- w235
          }
          frame 13 {
            n241 = property on="Color Box 28" class="ColBox"("Label.Visible"=FALSE) -> ()  [unwired: 2 in, 2 out]
            n242 = property on="Color Box 28" class="ColBox"("Visible"=TRUE) -> ()  [unwired: 2 in, 2 out]
            "Color Box 28" <- w238
          }
          frame 14 {
            n243 = property on="Color Box 29" class="ColBox"("Label.Visible"=FALSE) -> ()  [unwired: 2 in, 2 out]
            n244 = property on="Color Box 29" class="ColBox"("Visible"=TRUE) -> ()  [unwired: 2 in, 2 out]
            "Color Box 29" <- w241
          }
          frame 15 {
            n245 = property on="Color Box 30" class="ColBox"("Label.Visible"=FALSE) -> ()  [unwired: 2 in, 2 out]
            n246 = property on="Color Box 30" class="ColBox"("Visible"=TRUE) -> ()  [unwired: 2 in, 2 out]
            "Color Box 30" <- w244
          }
        }
      }
      n247 = while {
        stop <- w15 stop-if-true
        n248 = local read "Start"() -> (w13:bool)
        n249 = case shown="True" w13 {
          frame False {
          }
          frame True {
            n250 = property on="element" class="ColBox"("Visible"=TRUE) -> ()  [unwired: 2 in, 2 out]
            n251 = for {
              N: 600 -> [_]
              shift-right: [w23] -> _
              shift-left: 720 -> [w24]
              stop <- w22 stop-if-true
              n252 = Increment(x=w24) -> (x+1=w23:i32)
              n253 = property on="element" class="ColBox"("Left"=w23) -> ()  [unwired: 2 in, 2 out]
              n254 = local read "stop"() -> (w22:bool)
              n255 = property on="element" class="ColBox"("Label.Visible"=FALSE ("Visible")) -> ()  [unwired: 2 in, 2 out]
            }
            n256 = local write "Koniec przejazdu"(FALSE ("Koniec przejazdu")) -> ()
            "Przejazd na przenośniku" <- TRUE ("Visible")
          }
        }
        n257 = local read "stop"() -> (w15:bool)
        n258 = Wait (ms)(milliseconds to wait="milliseconds to wait 2") -> ()  [unwired: 1 out]
      }
    }
    frame #1 {
      n259 = property on="Color Box 6" class="ColBox"("Visible"=FALSE) -> ()  [unwired: 2 in, 2 out]
      n260 = property on="Color Box 20" class="ColBox"("Visible"=FALSE) -> ()  [unwired: 2 in, 2 out]
      n261 = property on="Color Box 31" class="ColBox"("Visible"=FALSE) -> ()  [unwired: 2 in, 2 out]
      n262 = property on="Color Box 24" class="ColBox"("Visible"=FALSE) -> ()  [unwired: 2 in, 2 out]
      n263 = property on="Color Box 35" class="ColBox"("Visible"=FALSE) -> ()  [unwired: 2 in, 2 out]
      n264 = property on="Color Box 28" class="ColBox"("Visible"=FALSE) -> ()  [unwired: 2 in, 2 out]
      n265 = property on="Color Box 39" class="ColBox"("Visible"=FALSE) -> ()  [unwired: 2 in, 2 out]
      n266 = property on="Color Box" class="ColBox"("Visible"=FALSE) -> ()  [unwired: 2 in, 2 out]
      n267 = property on="Color Box 43" class="ColBox"("Visible"=FALSE) -> ()  [unwired: 2 in, 2 out]
      n268 = property on="Color Box 5" class="ColBox"("Visible"=FALSE) -> ()  [unwired: 2 in, 2 out]
      n269 = property on="Color Box 10" class="ColBox"("Visible"=FALSE) -> ()  [unwired: 2 in, 2 out]
      n270 = property on="Color Box 15" class="ColBox"("Visible"=FALSE) -> ()  [unwired: 2 in, 2 out]
      n271 = property on="element" class="ColBox"("Visible"=FALSE) -> ()  [unwired: 2 in, 2 out]
      n272 = property on="element2" class="ColBox"("Visible"=FALSE) -> ()  [unwired: 2 in, 2 out]
      n273 = call <vilib>:"Disconnect.vi"("error in (no error)"=w364, "OPC UA client refnum in"=w363) -> ()  [unwired: 9 in, 1 out]
      n274 = property on="Color Box 12" class="ColBox"("Visible"=FALSE) -> ()  [unwired: 2 in, 2 out]
      n275 = property on="Color Box 21" class="ColBox"("Visible"=FALSE) -> ()  [unwired: 2 in, 2 out]
      n276 = property on="Color Box 32" class="ColBox"("Visible"=FALSE) -> ()  [unwired: 2 in, 2 out]
      n277 = property on="Color Box 36" class="ColBox"("Visible"=FALSE) -> ()  [unwired: 2 in, 2 out]
      n278 = property on="Color Box 25" class="ColBox"("Visible"=FALSE) -> ()  [unwired: 2 in, 2 out]
      n279 = property on="Color Box 2" class="ColBox"("Visible"=FALSE) -> ()  [unwired: 2 in, 2 out]
      n280 = property on="Color Box 29" class="ColBox"("Visible"=FALSE) -> ()  [unwired: 2 in, 2 out]
      n281 = property on="Color Box 40" class="ColBox"("Visible"=FALSE) -> ()  [unwired: 2 in, 2 out]
      n282 = property on="Color Box 7" class="ColBox"("Visible"=FALSE) -> ()  [unwired: 2 in, 2 out]
      n283 = property on="Color Box 44" class="ColBox"("Visible"=FALSE) -> ()  [unwired: 2 in, 2 out]
      n284 = property on="Color Box 11" class="ColBox"("Visible"=FALSE) -> ()  [unwired: 2 in, 2 out]
      n285 = property on="Color Box 16" class="ColBox"("Visible"=FALSE) -> ()  [unwired: 2 in, 2 out]
      n286 = local write "Przejazd na przenośniku"(FALSE ("Przejazd na przenośniku")) -> ()
      n287 = property on="Color Box 22" class="ColBox"("Visible"=FALSE) -> ()  [unwired: 2 in, 2 out]
      n288 = property on="Color Box 18" class="ColBox"("Visible"=FALSE) -> ()  [unwired: 2 in, 2 out]
      n289 = local write "Koniec przejazdu"(FALSE ("Koniec przejazdu")) -> ()
      n290 = property on="Color Box 37" class="ColBox"("Visible"=FALSE) -> ()  [unwired: 2 in, 2 out]
      n291 = property on="Color Box 33" class="ColBox"("Visible"=FALSE) -> ()  [unwired: 2 in, 2 out]
      n292 = property on="Color Box 26" class="ColBox"("Visible"=FALSE) -> ()  [unwired: 2 in, 2 out]
      n293 = property on="Color Box 41" class="ColBox"("Visible"=FALSE) -> ()  [unwired: 2 in, 2 out]
      n294 = property on="Color Box 8" class="ColBox"("Visible"=FALSE) -> ()  [unwired: 2 in, 2 out]
      n295 = property on="Color Box 3" class="ColBox"("Visible"=FALSE) -> ()  [unwired: 2 in, 2 out]
      n296 = property on="Color Box 30" class="ColBox"("Visible"=FALSE) -> ()  [unwired: 2 in, 2 out]
      n297 = property on="Color Box 13" class="ColBox"("Visible"=FALSE) -> ()  [unwired: 2 in, 2 out]
      n298 = property on="Color Box 45" class="ColBox"("Visible"=FALSE) -> ()  [unwired: 2 in, 2 out]
      n299 = property on="Color Box 17" class="ColBox"("Visible"=FALSE) -> ()  [unwired: 2 in, 2 out]
      n300 = local write "Praca robota"(FALSE ("Praca robota")) -> ()
      n301 = property on="Color Box 23" class="ColBox"("Visible"=FALSE) -> ()  [unwired: 2 in, 2 out]
      n302 = property on="Color Box 19" class="ColBox"("Visible"=FALSE) -> ()  [unwired: 2 in, 2 out]
      n303 = property on="Color Box 27" class="ColBox"("Visible"=FALSE) -> ()  [unwired: 2 in, 2 out]
      n304 = property on="Color Box 38" class="ColBox"("Visible"=FALSE) -> ()  [unwired: 2 in, 2 out]
      n305 = property on="Color Box 34" class="ColBox"("Visible"=FALSE) -> ()  [unwired: 2 in, 2 out]
      n306 = property on="Color Box 42" class="ColBox"("Visible"=FALSE) -> ()  [unwired: 2 in, 2 out]
      n307 = property on="Color Box 9" class="ColBox"("Visible"=FALSE) -> ()  [unwired: 2 in, 2 out]
      n308 = property on="Color Box 4" class="ColBox"("Visible"=FALSE) -> ()  [unwired: 2 in, 2 out]
      n309 = property on="Color Box 14" class="ColBox"("Visible"=FALSE) -> ()  [unwired: 2 in, 2 out]
      "Ilość elementów w koszu" <- 0.0 ("Ilość elementów w koszu")
      "Ilość elementów na palecie 3" <- 0.0 ("Ilość elementów na palecie 3")
      "Ilość elementów na palecie 2" <- 0.0 ("Ilość elementów na palecie 2")
      "Ilość elementów na palecie 1" <- 0.0 ("Ilość elementów na palecie 1")
      "Wrzucanie do kosza" <- FALSE ("Wrzucanie do kosza")
      "Układanie na palecie 1" <- FALSE ("Układanie na palecie 1")
      "Układanie na palecie 2" <- FALSE ("Układanie na palecie 2")
      "Układanie na palecie 3" <- FALSE ("Układanie na palecie 3")
    }
  }
